vi "SPI Configure.vi"(8 "Error In":errorcluster, 9 "SPI Configuration":T1, 10 "SPI Channel":u8, 11 "LINX Resource":T6) -> (0 "Error Out":errorcluster, 3 "LINX Resource":T6)   [LabVIEW 2011, in "LVH-LINX.lvlib"]
doc: "Configure the specified SPI channel."
uses:
  LVH-LINX.lvlib
  Private/Type Defs/LINX Ref.ctl
  Private/Type Defs/Platform.ctl
  Private/Type Defs/Interface.ctl
  Private/Device/Type Defs/LINX Device Config.ctl
  Private/Device/Type Defs/TCP Config.ctl
  Private/Type Defs/Device Family.ctl
  Private/Type Defs/Peripherals/SPI/SPI Configuration.ctl
  Private/Type Defs/Peripherals/SPI/SPI Bit Order.ctl
  Private/Type Defs/Peripherals/SPI/SPI Clock Phase.ctl
  Private/Type Defs/Peripherals/SPI/SPI Clock Polarity.ctl
  Private/Type Defs/Peripherals/SPI/SPI CS Logic Level.ctl
  Private/Type Defs/Peripheral.ctl
  Private/Type Defs/Channel FGV States.ctl
  Private/Device/Device.lvlib
  <vilib>/myRIO/Common/Instrument Driver Framework/myRIO v1.0/SPI/typedefs/SPI Frame Length.ctl
  <vilib>/myRIO/Common/Instrument Driver Framework/myRIO v1.0/SPI/typedefs/SPI Data Direction.ctl
  <vilib>/myRIO/Common/Instrument Driver Framework/myRIO v1.0/SPI/typedefs/SPI Clock Polarity.ctl
  <vilib>/myRIO/Common/Instrument Driver Framework/myRIO v1.0/SPI/typedefs/SPI Clock Phase.ctl
  <vilib>/myRIO/Instrument Drivers/Onboard IO/SPI/typedefs/SPI Configuration.ctl
  <vilib>/myRIO/Common/Instrument Driver Framework/myRIO v1.0/SPI/typedefs/SPI Channels Enum.ctl
  <vilib>/myRIO/Common/Instrument Driver Framework/Utilities/typedefs/Generic FPGA Reference.ctl
  <vilib>/myRIO/Common/Instrument Driver Framework/Utilities/typedefs/myRIO v1.0 Reference.ctl
  <vilib>/myRIO/Common/Instrument Driver Framework/Utilities/typedefs/Hardware Version Enum.ctl
  <vilib>/myRIO/Common/Instrument Driver Framework/Utilities/typedefs/myRIO Generic Hardware Reference.ctl
  <vilib>/myRIO/Instrument Drivers/Onboard IO/SPI/typedefs/SPI Reference.ctl
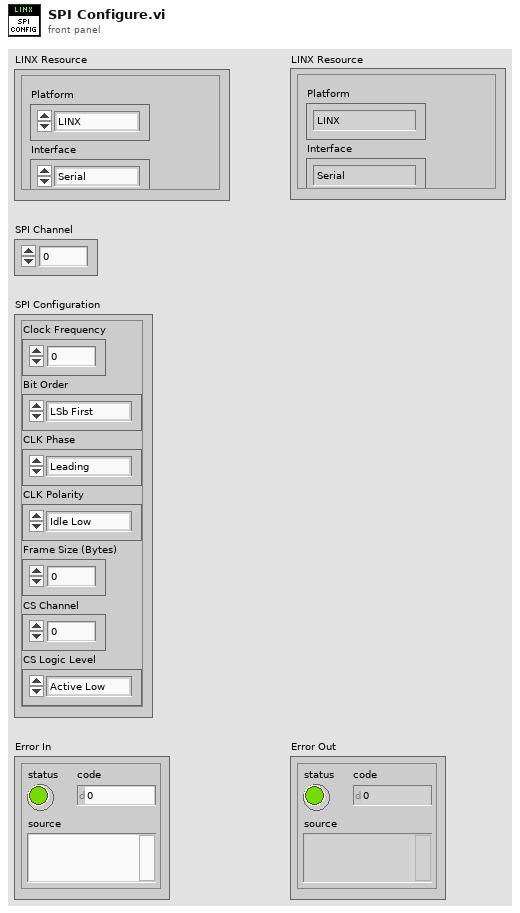
[diagram p1: front panel]
types:
  T1 = typedef "LVH-LINX.lvlib/SPI Configuration.ctl" = cluster{"Clock Frequency":u32, "Bit Order":T2, "CLK Phase":T3, "CLK Polarity":T4, "Frame Size (Bytes)":u8, "CS Channel":u8, "CS Logic Level":T5}
  T2 = typedef "LVH-LINX.lvlib/SPI Bit Order.ctl" = enum8{"LSb First", "MSb First"}
  T3 = typedef "LVH-LINX.lvlib/SPI Clock Phase.ctl" = enum8{"Leading", "Trailing"}
  T4 = typedef "LVH-LINX.lvlib/SPI Clock Polarity.ctl" = enum8{"Idle Low", "Idle High"}
  T5 = typedef "LVH-LINX.lvlib/SPI CS Logic Level.ctl" = enum8{"Active Low", "Active High"}
  T6 = typedef "LVH-LINX.lvlib/LINX Ref.ctl" = cluster{"Platform":T7, "Interface":T8, "LINX Device Config":T9}
  T7 = typedef "LVH-LINX.lvlib/Platform.ctl" = enum16{"LINX", "myRIO"}
  T8 = typedef "LVH-LINX.lvlib/Interface.ctl" = enum16{"Serial", "TCP"}
  T9 = typedef "LVH-LINX.lvlib/Device.lvlib/LINX Device Config.ctl" = cluster{"Interface":T8, "COM Port":refnum<visa-resource-name>, "TCP Configuration":T10, "Device Family":T11, "Device ID":u8, "Device Name":string, "TCP Ref":refnum<k5>}
  T10 = typedef "LVH-LINX.lvlib/Device.lvlib/TCP Config.ctl" = cluster{"IP Address":string, "Port":u16}
  T11 = typedef "LVH-LINX.lvlib/Device Family.ctl" = enum8{"National Instruments", "Digilent", "Arduino"}
  T12 = typedef "LVH-LINX.lvlib/Peripheral.ctl" = enum8{"DI", "DO", "AI", "AO", "PWM", "QE", "UART", "I2C", "SPI", "CAN"}
  T13 = cluster{"Frequency":dbl, "Clock Phase":u8, "Clock Polarity":u8, "Data Direction":u8, "Frame Length":u8}
  T14 = typedef "LVH-LINX.lvlib/Channel FGV States.ctl" = enum16{"Initialize", "Get", "Set"}
  T15 = typedef "SPI.lvlib/SPI Reference.ctl" = cluster{"myRIO Reference":T16, "SPI Channels Enum":T20, "SPI Configuration":T21}
  T16 = typedef "myRIO Generic Hardware Reference.ctl" = cluster{"myRIO Model":T17, "myRIO Hardware Reference":T18}
  T17 = typedef "Hardware Version Enum.ctl" = enum16{"Unknown", "myRIO-1900", "myRIO-1950"}
  T18 = typedef "myRIO v1.0 Reference.ctl" = cluster{"Generic FPGA Reference":T19, "Allow multiple opens":bool}
  T19 = typedef "Generic FPGA Reference.ctl" = refnum<k20>
  T20 = typedef "SPI Channels Enum.ctl" = enum16{"Not Connected", "A/SPI", "B/SPI"}
  T21 = typedef "SPI.lvlib/SPI Configuration.ctl" = cluster{"Frequency (Hz)":dbl, "Clock Phase":T22, "Clock Polarity":T23, "Data Direction":T24, "Frame Length":T25}
  T22 = typedef "SPI Clock Phase.ctl" = enum8{"Leading", "Trailing"}
  T23 = typedef "SPI Clock Polarity.ctl" = enum8{"Low", "High"}
  T24 = typedef "SPI Data Direction.ctl" = enum8{"Most Significant Bit First", "Least Significant Bit First"}
  T25 = typedef "SPI Frame Length.ctl" = u8
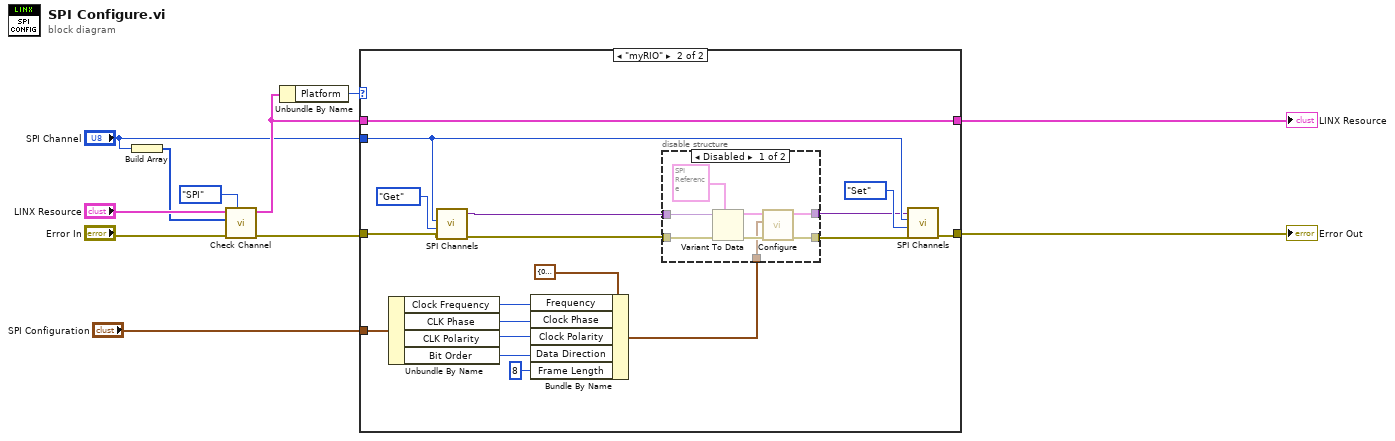
[diagram p0: block diagram]
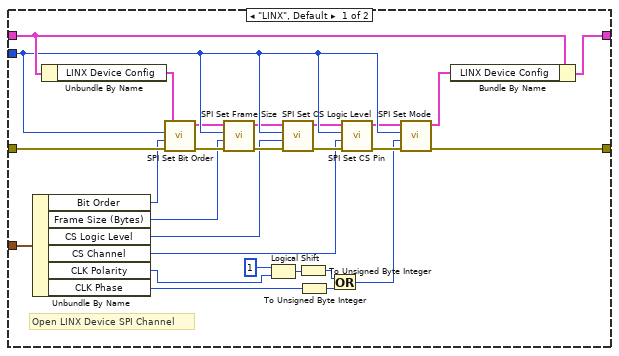
[diagram p2: hidden frame]
diagram:
  n1 = Build Array("SPI Channel") -> (w4:u8[])
  n2 = call "Check Channel.vi"("Peripheral"=Peripheral."SPI", "Error In"="Error In", "Channels"=w4, "LINX Resource"="LINX Resource") -> ("Error Out"=w5:errorcluster, "LINX Resource"=w6:T6)  [unwired: 5 in, 1 out]
  n3 = Unbundle By Name(w6) -> ("Platform"=w11:T7)
  n4 = case shown="\"myRIO\"" w11 {
    tunnel: w5 -> [w30 w53]
    tunnel: w6 -> [w38 w56]
    tunnel: [w12 w55] -> w10
    tunnel: [w37 w56] -> w9
    tunnel: "SPI Channel" -> [w35 w52]
    tunnel: "SPI Configuration" -> [w24 w50]
    frame "LINX", Default {
      # "Open LINX Device SPI Channel"
      n5 = Unbundle By Name(w24) -> ("Bit Order"=w23:T2, "Frame Size (Bytes)"=w22:u8, "CS Logic Level"=w21:T5, "CS Channel"=w20:u8, "CLK Polarity"=w19:T4, "CLK Phase"=w15:T3)
      n6 = Unbundle By Name(w38) -> ("LINX Device Config"=w36:T9)
      n7 = call "SPI Set Bit Order.vi"("Error In"=w30, "SPI Bit Order"=w23, "SPI Channel"=w35, "LINX Device Config"=w36) -> ("Error Out"=w29:errorcluster, "LINX Device Config"=w34:T9)  [unwired: 6 in]
      n8 = call "SPI Set Frame Size.vi"("Error In"=w29, "Frame Size (Bytes)"=w22, "SPI Channel"=w35, "LINX Device Config"=w34) -> ("Error Out"=w27:errorcluster, "LINX Device Config"=w33:T9)  [unwired: 6 in]
      n9 = Logical Shift(y=u8 1, x=w19) -> (x << y=w18:u32)
      n10 = call "SPI Set CS Logic Level.vi"("Error In"=w27, "CS Logic Level"=w21, "SPI Channel"=w35, "LINX Device Config"=w33) -> ("Error Out"=w28:errorcluster, "LINX Device Config"=w32:T9)  [unwired: 6 in]
      n11 = To Unsigned Byte Integer(number=w18) -> (unsigned 8bit integer=w17:u8)
      n12 = To Unsigned Byte Integer(number=w15) -> (unsigned 8bit integer=w16:u8)
      n13 = Or(x=w17, y=w16) -> (x .or. y?=w14:u8)
      n14 = call "SPI Set CS Pin.vi"("Error In"=w28, "CS Pin"=w20, "SPI Channel"=w35, "LINX Device Config"=w32) -> ("Error Out"=w26:errorcluster, "LINX Device Config"=w31:T9)  [unwired: 6 in]
      n15 = call "SPI Set Mode.vi"("Error In"=w26, "Mode"=w14, "SPI Channel"=w35, "LINX Device Config"=w31) -> ("Error Out"=w12:errorcluster, "LINX Device Config"=w13:T9)  [unwired: 6 in]
      n16 = Bundle By Name(cluster=w38, "LINX Device Config"=w13) -> (w37:T6)
    }
    frame "myRIO" {
      n17 = Unbundle By Name(w50) -> ("Clock Frequency"=w46:u32, "CLK Phase"=w44:T3, "CLK Polarity"=w43:T4, "Bit Order"=w42:T2)
      n18 = call "SPI Channels.vi"("Error In"=w53, "Channel State"=Channel_FGV_States."Get", "Channel Number"=w52) -> ("Error Out"=w49:errorcluster, "SPI Channel"=w40:variant)  [unwired: 7 in]
      n19 = Bundle By Name(cluster=T13 {"Frequency"=0.0, "Clock Phase"=0, "Clock Polarity"=0, "Data Direction"=0, "Frame Length"=0}, "Frequency"=w46, "Clock Phase"=w44, "Clock Polarity"=w43, "Data Direction"=w42, "Frame Length"=u8 8) -> (w39:T13)
      n20 = disable-structure shown="Disabled" {
        disable-tunnel: w49 -> [w61 _]
        disable-tunnel: [w60 _] -> w48
        disable-tunnel: [w59 _] -> w41
        disable-tunnel: w40 -> [w58 _]
        disable-tunnel: w39 -> [w57 _]
        frame Disabled {
          n21 = Variant To Data(error in=w61, type=T15 {"myRIO Reference"={"myRIO Model"=enum."Unknown", "myRIO Hardware Reference"={"Generic FPGA Reference"=refnum, "Allow multiple opens"=FALSE}}, "SPI Channels Enum"=enum."Not Connected", "SPI Configuration"={"Frequency (Hz)"=0.0, "Clock Phase"=enum."Leading", "Clock Polarity"=enum."Low", "Data Direction"=enum."Most Significant Bit First", "Frame Length"=8}} ("SPI Ref In"), Variant=w58) -> (data=w63:T15, error out=w62:errorcluster)
          n22 = call <vilib>:"Configure.vi"("error in (no error)"=w62, "SPI User Configuration"=w57, "SPI Ref In"=w63) -> ("error out"=w60:errorcluster, "SPI Ref Out"=w59:T15)  [unwired: 7 in]
        }
        frame Enabled {
        }
      }
      n23 = call "SPI Channels.vi"("Error In"=w48, "Channel State"=Channel_FGV_States."Set", "Channel Number"=w52, "SPI Channel"=w41) -> ("Error Out"=w55:errorcluster)  [unwired: 6 in, 1 out]
    }
  }
  "Error Out" <- w10
  "LINX Resource" <- w9
